vi "COnfigAuto.vi"(8 "Remote 2 Nodes":T2={"button 1"=TRUE, "button 2"=TRUE, "button 3"=TRUE, "button 4"=TRUE, "button 5"=TRUE, "button 6"=TRUE, "button 7"=TRUE, "button 8"=TRUE, "button 9"=TRUE, "button 10"=TRUE, "button 11"=TRUE, "button 12"=TRUE, "POV"=TRUE, "Left X"=TRUE, "Left Y"=TRUE, "Right X"=TRUE, "Right Y"=TRUE}, 9 "Remote 1 Nodes":T2={"button 1"=TRUE, "button 2"=TRUE, "button 3"=TRUE, "button 4"=TRUE, "button 5"=TRUE, "button 6"=TRUE, "button 7"=TRUE, "button 8"=TRUE, "button 9"=TRUE, "button 10"=TRUE, "button 11"=TRUE, "button 12"=TRUE, "POV"=TRUE, "Left X"=TRUE, "Left Y"=TRUE, "Right X"=TRUE, "Right Y"=TRUE}, 11 "NXT":T1={"Hardware"="NXT", "Flattened String"=""}) -> (3 "NXT":T1={"Hardware"="NXT", "Flattened String"=""})   [LabVIEW 2010, in "Packet Recorder.lvlib"]
uses:
  Packet Recorder.lvlib
  ConfigData.ctl
  <vilib>/NXT/Subs/LVHSConnector.ctl
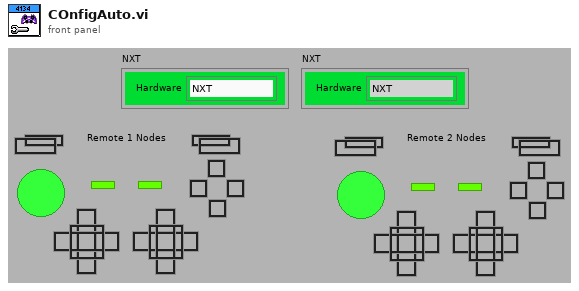
[diagram p1: front panel]
types:
  T1 = typedef "LVHSConnector.ctl" = cluster{"Hardware":string, "Flattened String":string}
  T2 = typedef "Packet Recorder.lvlib/ConfigData.ctl" = cluster{"button 1":bool, "button 2":bool, "button 3":bool, "button 4":bool, "button 5":bool, "button 6":bool, "button 7":bool, "button 8":bool, "button 9":bool, "button 10":bool, "button 11":bool, "button 12":bool, "POV":bool, "Left X":bool, "Left Y":bool, "Right X":bool, "Right Y":bool}
  T3 = cluster{"B1-12:B1-12:POV1-4:POV1-4":bool[], "1LXY:RXY:2LXY:RXY":bool[]}
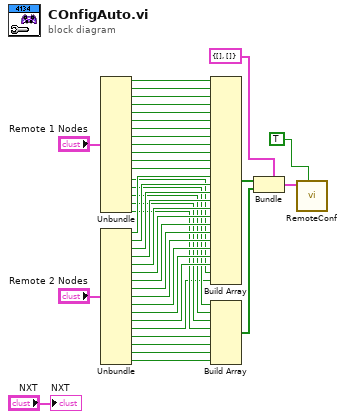
[diagram p0: block diagram]
diagram:
  n1 = Unbundle("Remote 1 Nodes") -> ("button 1"=w28:bool, "button 2"=w29:bool, "button 3"=w30:bool, "button 4"=w31:bool, "button 5"=w32:bool, "button 6"=w33:bool, "button 7"=w34:bool, "button 8"=w35:bool, "button 9"=w36:bool, "button 10"=w37:bool, "button 11"=w38:bool, "button 12"=w39:bool, "POV"=w15:bool, "Left X"=w14:bool, "Left Y"=w13:bool, "Right X"=w12:bool, "Right Y"=w11:bool)
  n2 = Unbundle("Remote 2 Nodes") -> ("button 1"=w27:bool, "button 2"=w26:bool, "button 3"=w25:bool, "button 4"=w24:bool, "button 5"=w23:bool, "button 6"=w22:bool, "button 7"=w21:bool, "button 8"=w20:bool, "button 9"=w19:bool, "button 10"=w18:bool, "button 11"=w17:bool, "button 12"=w16:bool, "POV"=w1:bool, "Left X"=w10:bool, "Left Y"=w9:bool, "Right X"=w8:bool, "Right Y"=w7:bool)
  n3 = Build Array(w28, w29, w30, w31, w32, w33, w34, w35, w36, w37, w38, w39, w27, w26, w25, w24, w23, w22, w21, w20, w19, w18, w17, w16, w15, w1) -> (w5:bool[])
  n4 = Build Array(w14, w13, w12, w11, w10, w9, w8, w7) -> (w6:bool[])
  n5 = Bundle(cluster=T3 {"B1-12:B1-12:POV1-4:POV1-4"=[], "1LXY:RXY:2LXY:RXY"=[]}, "B1-12:B1-12:POV1-4:POV1-4"=w5, "1LXY:RXY:2LXY:RXY"=w6) -> (w3:T3)
  n6 = call "RemoteConf.vi"("Write?"=TRUE, "ConfInput"=w3) -> ()  [unwired: 9 in, 1 out]
  "NXT" <- "NXT"
